vi "VB MIDI AM Gen.vi"() -> ()   [LabVIEW 2018]
uses:
  MessageTD.ctl
  <vilib>/measure/NI_MABase.lvlib
panel:
  out "AM Output":waveform(dbl)[](graph)
  out "ModulationWave":waveform(dbl)[](graph)
  out "CarrierWave":waveform(dbl)[](graph)
  out "FFTWave":cluster{"f0":dbl, "df":dbl, "magnitude":dbl[]}[](graph)
  in  "ModulationAmp":dbl=1.0 format="%0.2f"
  in  "CarrierFre":dbl=0.0078125 format="%0.4e"
  in  "CarrierAmp":dbl=1.0 format="%0.2f"
  in  "File Path":path
  in  "Play Button":bool
  in  "error in":errorcluster
  out "error out":errorcluster
  in  "VirtualBench \nDevice Handle":tag caption="Device Name"
  in  "Stop":bool
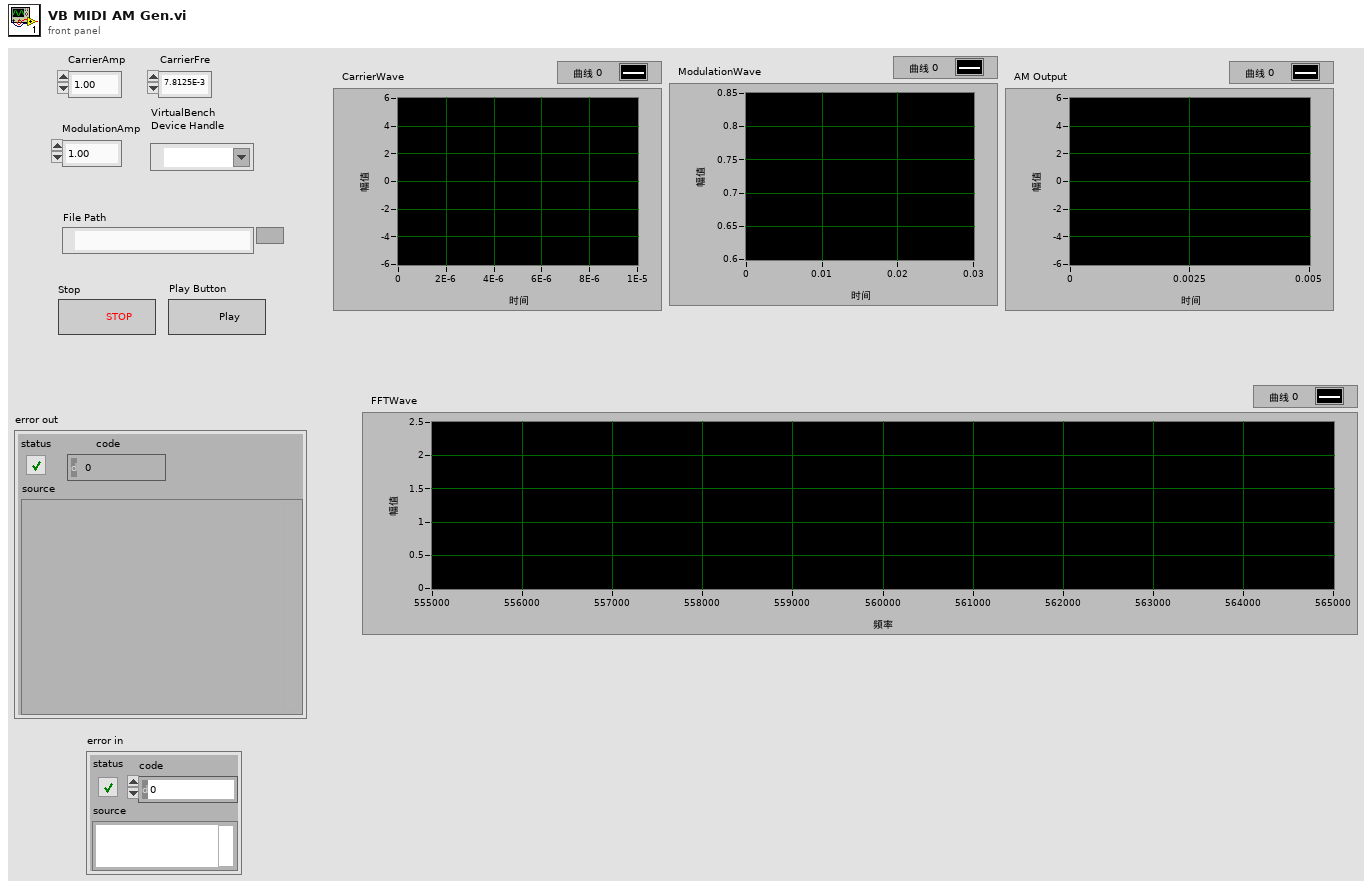
[diagram p1: front panel]
types:
  T1 = typedef "MessageTD.ctl" = enum16{"Idle", "Initialize", "Play", "Stop"}
  T2 = cluster{"Array of Waveform":waveform(dbl)[], waveform(dbl)[], waveform(dbl)[]}
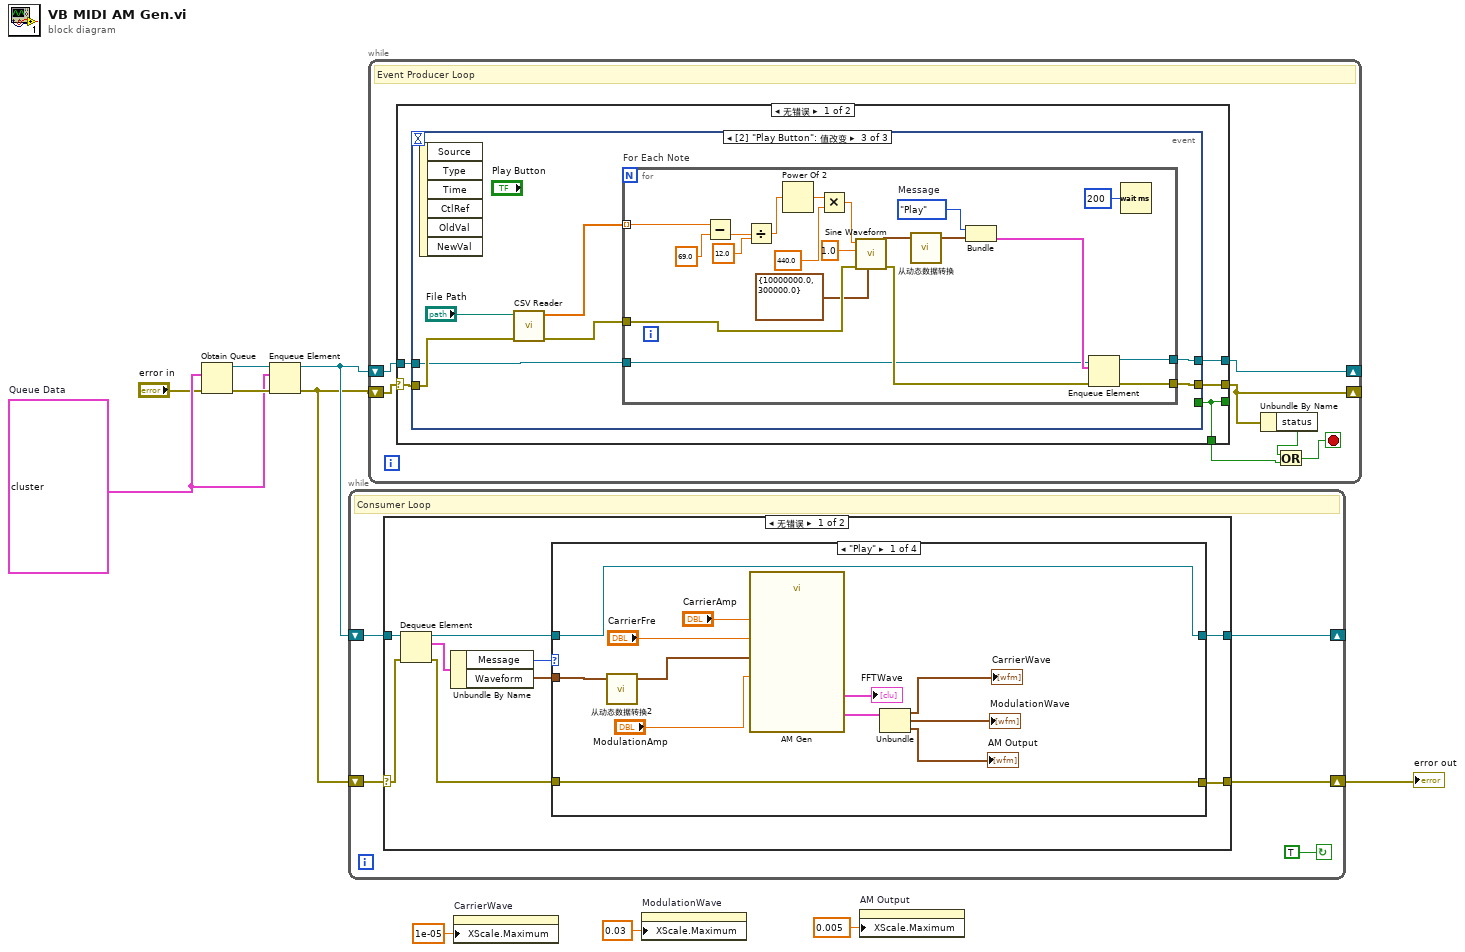
[diagram p0: block diagram]
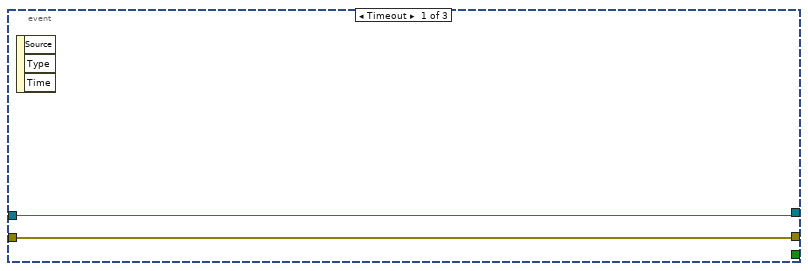
[diagram p2: hidden frame]
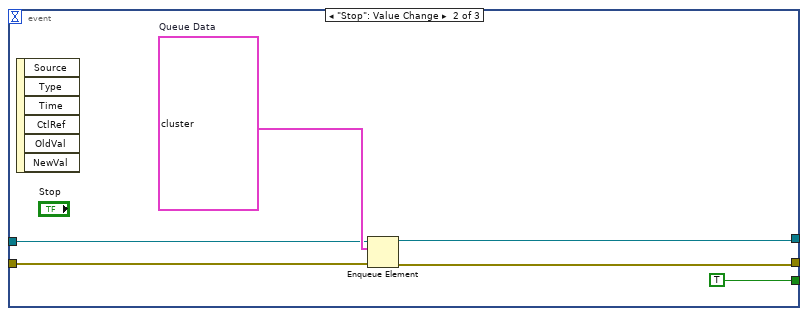
[diagram p3: hidden frame]
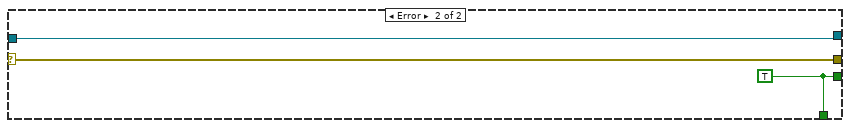
[diagram p4: hidden frame]
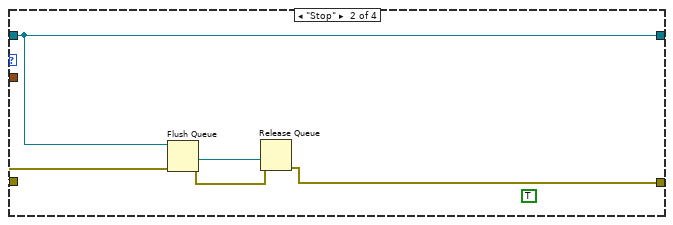
[diagram p5: hidden frame]
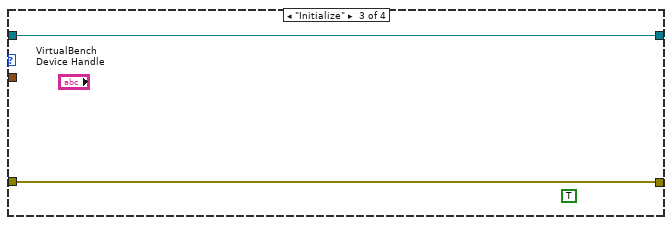
[diagram p6: hidden frame]
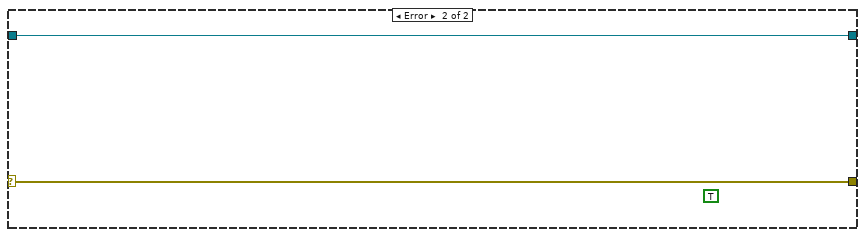
[diagram p8: hidden frame]
diagram:
  w8 = cluster{"Message":T1, "Waveform":waveform(dbl)} {"Message"=enum."Initialize", "Waveform"={"t0"=timestamp(0 s since 1904-01-01), "dt"=1.0, "Y"=[]}}  # Queue Data
  n1 = Obtain Queue(element data type=w8, error in (no error)="error in") -> (queue out=w9:refnum<queue>, error out=w10:errorcluster)  [unwired: 3 in, 1 out]
  n2 = Enqueue Element(queue=w9, element=w8, error in (no error)=w10) -> (queue out=w5:refnum<queue>, error out=w4:errorcluster)  [unwired: 1 in, 1 out]
  n3 = while {
    shift-right: [w14] -> w6
    shift-left: w4 -> [w12]
    shift-right: [w13] -> _
    shift-left: w5 -> [w15]
    stop <- TRUE ("y") continue-if-true
    # "Consumer Loop"
    n4 = case shown="无错误" w12 {
      selector: w12 -> [w18 w46]
      tunnel: w15 -> [w24 w47]
      tunnel: [w16 w46] -> w14
      tunnel: [w17 w47] -> w13
      frame No Error {
        n5 = Dequeue Element(queue=w24, error in (no error)=w18) -> (queue out=w19:refnum<queue>, element=w23:cluster{"Message":T1, "Waveform":waveform(dbl)}, error out=w21:errorcluster)  [unwired: 1 in, 1 out]
        n6 = Unbundle By Name(w23) -> ("Message"=w22:T1, "Waveform"=w20:waveform(dbl))
        n7 = case shown="\"Play\"" w22 {
          tunnel: w21 -> [w30 w40 w42 w44]
          tunnel: w20 -> [w33 _ _ _]
          tunnel: w19 -> [w29 w37 w43 w45]
          tunnel: [w29 w37 w43 w45] -> w17
          tunnel: [w30 w39 w42 w44] -> w16
          frame "Play" {
            n8 = call "从动态数据转换2"("Dynamic Data Type"=w33) -> ("Array of Waveform"=w32:waveform(dbl)[])  [unwired: 3 in]
            n9 = call "AM Gen.vi"("MIDI Waveform"=w32, "ModulationAmp"="ModulationAmp", "CarrierFre"="CarrierFre", "CarrierAmp"="CarrierAmp") -> ("FFTWave"=→"FFTWave":cluster{"f0":dbl, "df":dbl, "magnitude":dbl[]}[], "输出簇"=w28:T2)  [unwired: 6 in]
            n10 = Unbundle(w28) -> ("Array of Waveform"=→"CarrierWave":waveform(dbl)[], →"ModulationWave":waveform(dbl)[], →"AM Output":waveform(dbl)[])
          }
          frame "Stop" {
            (unwired) TRUE
            n11 = Flush Queue(queue=w37, error in (no error)=w40) -> (queue out=w38:refnum<queue>, error out=w41:errorcluster)  [unwired: 1 out]
            n12 = Release Queue(queue=w38, error in (no error)=w41) -> (error out=w39:errorcluster)  [unwired: 1 in, 2 out]
          }
          frame "Initialize" {
            (unwired) TRUE
          }
          frame "Idle", Default {
          }
        }
      }
      frame Error {
        (unwired) TRUE
      }
    }
  }
  "error out" <- w6
  n13 = while {
    shift-right: [w50] -> _
    shift-left: w4 -> [w49]
    shift-right: [w51] -> _
    shift-left: w5 -> [w52]
    stop <- w53 stop-if-true
    # "Event Producer Loop"
    n14 = case shown="无错误" w49 {
      selector: w49 -> [w59 w96]
      tunnel: [w58 w95] -> _
      tunnel: [w58 w95] -> w54
      tunnel: [w57 w96] -> w50
      tunnel: [w56 w97] -> w51
      tunnel: w52 -> [w55 w97]
      frame No Error {
        n15 = event shown="[2] \"Play Button\": 值改变" {
          selector: _ -> [_ _ _]
          dyn-events: _ -> [_ _ _]
          timeout: _ -> [_ _ _]
          tunnel: w59 -> [w60 w65 w73]
          tunnel: [_ TRUE _] -> w58
          tunnel: [w60 w63 w71] -> w57
          tunnel: [w61 w64 w70] -> w56
          tunnel: w55 -> [w61 w62 w69]
          event Timeout {
            n16 = event-data() -> ()  [unwired: 1 in, 3 out]
          }
          event "Stop": Value Change {
            w66 = cluster{"Message":T1, "Waveform":waveform(dbl)} {"Message"=enum."Initialize", "Waveform"={"t0"=timestamp(0 s since 1904-01-01), "dt"=1.0, "Y"=[]}}  # Queue Data
            n17 = event-data() -> ()  [unwired: 1 in, 6 out]
            n18 = Enqueue Element(queue=w62, element=w66, error in (no error)=w65) -> (queue out=w64:refnum<queue>, error out=w63:errorcluster)  [unwired: 1 in, 1 out]
          }
          event "Play Button": Value Change {
            n19 = event-data() -> ()  [unwired: 1 in, 6 out]
            n20 = call "CSV Reader.vi"("error in"=w73, "file (use dialog)"="File Path") -> ("error out"=w72:errorcluster, "Notes Array"=w68:dbl[])  [unwired: 8 in]
            n21 = for "For Each Note" {
              tunnel: [w85] -> w70
              tunnel: w72 -> [w82]
              tunnel: [w81] -> w71
              tunnel: w69 -> [w79]
              tunnel: w68 -> [w77] mode=indexing
              w87 = MessageTD."Play"  # Message
              n22 = Subtract(x=w77, y=69.0) -> (x-y=w94:dbl)
              n23 = Divide(x=w94, y=12.0) -> (x/y=w76:dbl)
              n24 = Power Of 2(x=w76) -> (2^x=w75:dbl)
              n25 = Multiply(x=w75, y=440.0) -> (x*y=w90:dbl)
              n26 = call <vilib>:"Sine Waveform.vi"("sampling info"=cluster{"Fs":dbl, "#s":dbl} {"Fs"=10000000.0, "#s"=300000.0}, "error in (no error)"=w82, "amplitude"=1.0, "frequency"=w90) -> ("error out"=w84:errorcluster, "signal out"=w88:waveform(dbl))  [unwired: 6 in]
              n27 = call "从动态数据转换"("Dynamic Data Type"=w88) -> ("Waveform"=w86:waveform(dbl))  [unwired: 3 in]
              n28 = Bundle("Message"=w87, "Waveform"=w86) -> (w80:cluster{"Message":T1, "Waveform":waveform(dbl)})  [unwired: 1 in]
              n29 = Enqueue Element(queue=w79, element=w80, error in (no error)=w84) -> (queue out=w85:refnum<queue>, error out=w81:errorcluster)  [unwired: 1 in, 1 out]
              n30 = Wait (ms)(milliseconds to wait=u32 200 ("等待时间（毫秒）")) -> ()  [unwired: 1 out]
            }
          }
        }
      }
      frame Error {
        w95 = TRUE
      }
    }
    n31 = Unbundle By Name(w50) -> ("status"=w48:bool)
    n32 = Or(x=w48, y=w54) -> (x .or. y?=w53:bool)
  }
  n33 = property on="CarrierWave" class="WFGraph (严格)"("XScale.Maximum"=1e-05 ("X标尺.范围:最大值")) -> ()  [unwired: 2 in, 2 out]
  n34 = property on="ModulationWave" class="WFGraph (严格)"("XScale.Maximum"=0.03 ("X标尺.范围:最大值")) -> ()  [unwired: 2 in, 2 out]
  n35 = property on="AM Output" class="WFGraph (严格)"("XScale.Maximum"=0.005 ("X标尺.范围:最大值")) -> ()  [unwired: 2 in, 2 out]
